vi "generateTimeString.vi"(10 "time vector":dbl[](array[numeric])) -> (2 "time":string)   [LabVIEW 2010]
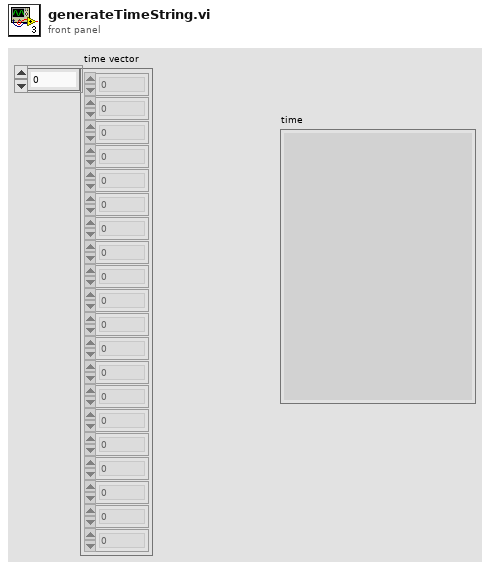
[diagram p1: front panel]
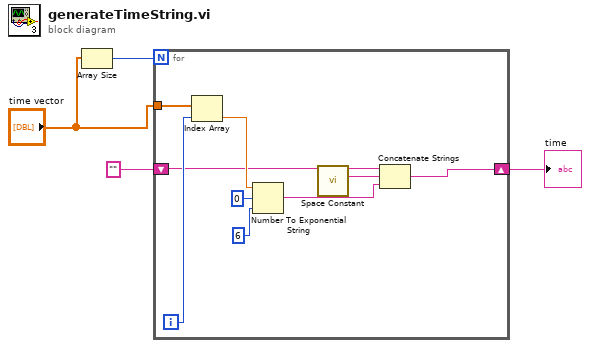
[diagram p0: block diagram]
diagram:
  n1 = Array Size(array="time vector") -> (size(s)=w4:i32)
  n2 = for {
    N: w4 -> [_]
    shift-right: [w13] -> w2
    shift-left: "" -> [w8]
    tunnel: "time vector" -> [w12]
    i -> [w10]
    n3 = Index Array(array=w12, index=w10) -> (element=w11:dbl)
    n4 = Number To Exponential String(number=w11, precision (6)=i16 6, 3:i16 0 ("width (-)")) -> (E-format string=w9:string)  [unwired: 1 in]
    n5 = call <vilib>:"Space Constant.vi"() -> ("String"=w5:string)
    n6 = Concatenate Strings(w8, w5, w9) -> (w13:string)
  }
  "time" <- w2
